vi "Get Channel DC Offset.vi"(8 "error in (no error)":errorcluster, 10 "Params":variant, 11 "PI650 VoltageAmp in":refnum<class "PI650 VoltageAmp.lvclass">) -> (0 "error out":errorcluster, 2 "Value":variant, 3 "PI650 VoltageAmp out":refnum<class "PI650 VoltageAmp.lvclass">)   [LabVIEW 2020, in "Pickering.lvlib" / "PI650 VoltageAmp.lvclass"]
uses:
  PI650 VoltageAmp.lvclass
  PI650 VoltageAmp.lvclass/PI650 VoltageAmp.ctl
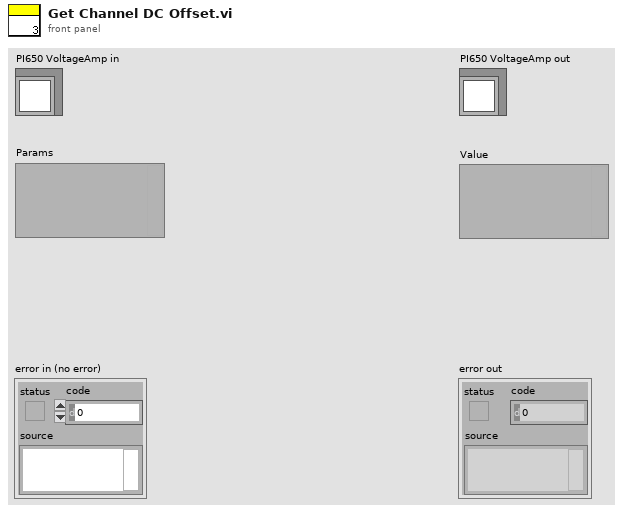
[diagram p1: front panel]
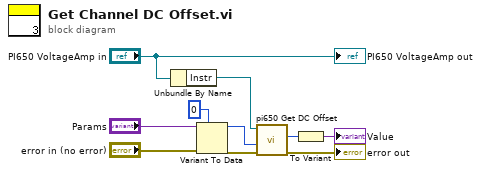
[diagram p0: block diagram]
diagram:
  n1 = Unbundle By Name("PI650 VoltageAmp in") -> ("Instr"=w9:refnum<visa-resource-name>)
  n2 = Variant To Data(error in="error in (no error)", type=u32 0 ("Channel (0)"), Variant="Params") -> (data=w5:u32, error out=w4:errorcluster)
  n3 = call <instrlib>:"pi650 Get DC Offset.vi"("error in (no error)"=w4, "Channel (0)"=w5, "instrument handle"=w9) -> ("error out"=→"error out":errorcluster, "Offset"=w2:u32)  [unwired: 6 in, 1 out]
  n4 = To Variant(anything=w2) -> (Variant=→"Value":variant)
  "PI650 VoltageAmp out" <- "PI650 VoltageAmp in"
